vi "TCP_TB.vi"(4 "IP ADDRESS":string="192.168.0.100", 5 "error in (no error)":errorcluster, 6 "COMMAND":string, 8 "Connection ID IN":refnum<k5>) -> (0 "error out":errorcluster, 2 "Decimal Number":u32, 3 "Their Response:":string)   [LabVIEW 2013]
panel:
  out "Connection ID IN 2":refnum<k5>
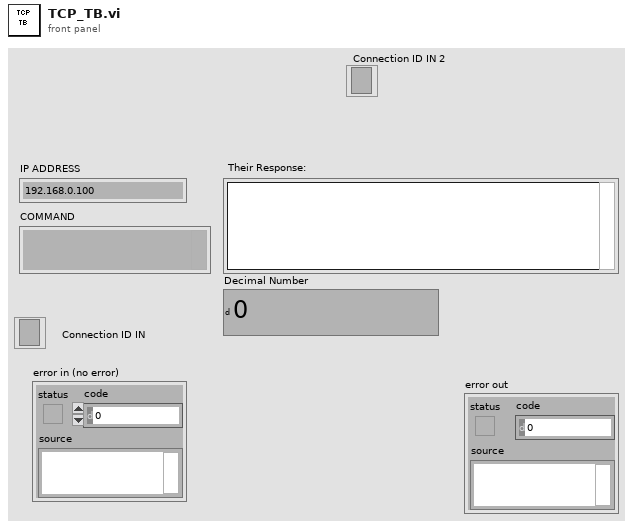
[diagram p1: front panel]
types:
  T1 = enum16{"Standard", "Buffered", "CRLF", "Immediate"}
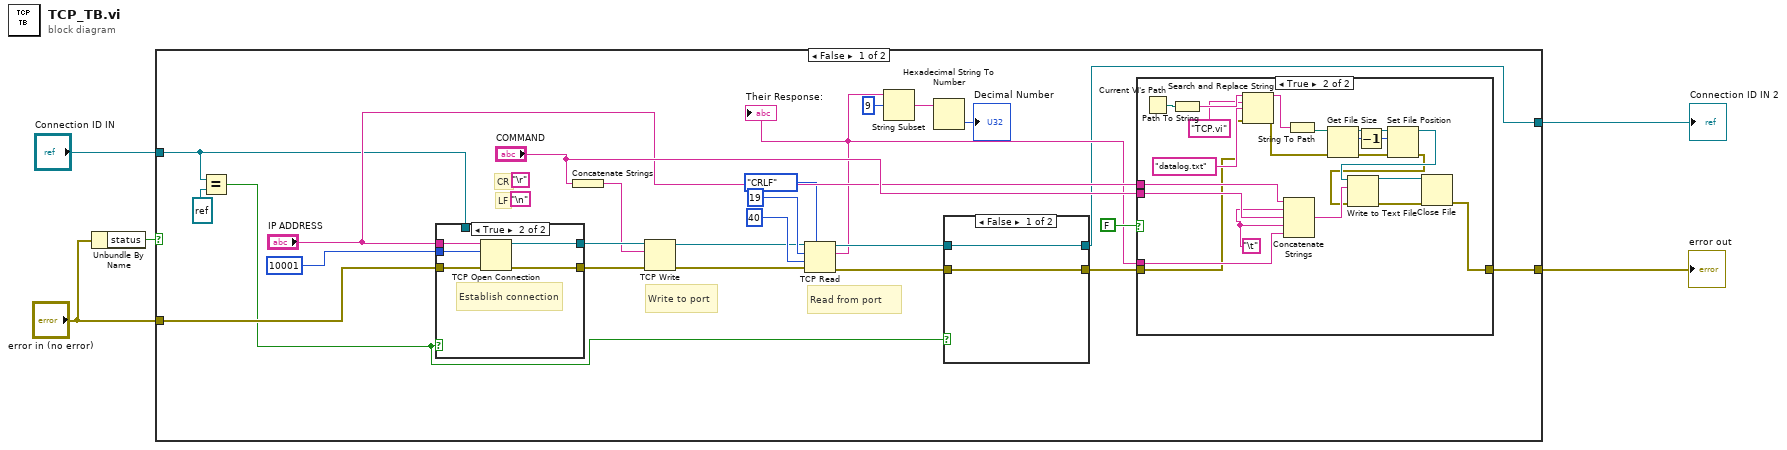
[diagram p0: block diagram]
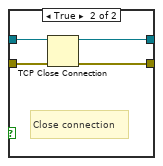
[diagram p3: hidden frame]
diagram:
  n1 = Unbundle By Name("error in (no error)") -> ("status"=w3:bool)
  n2 = case shown="False" w3 {
    tunnel: [w18 w68] -> w5
    tunnel: "error in (no error)" -> [w17 w68]
    tunnel: "Connection ID IN" -> [w9 w67]
    tunnel: [w6 w67] -> w1
    frame False {
      (unwired) "\n"
      (unwired) "\r"
      # "Read from port"
      # "Write to port"
      # "LF"
      # "CR"
      n3 = Equal?(x=w9, y=refnum<k5> refnum ("connection ID")) -> (x = y?=w7:bool)
      n4 = case shown="True" w7 {
        tunnel: [w31 w37] -> w27
        tunnel: [w32 w36] -> w26
        tunnel: u16 10001 ("remote port") -> [_ w35]
        tunnel: "IP ADDRESS" -> [_ w34]
        tunnel: w17 -> [w31 w33]
        tunnel: w9 -> [w32 _]
        frame False {
        }
        frame True {
          # "Establish connection"
          n5 = TCP Open Connection(address=w34, remote port or service name=w35, error in (no error)=w33) -> (connection ID=w36:refnum<k5>, error out=w37:errorcluster)  [unwired: 2 in]
        }
      }
      n6 = Concatenate Strings("COMMAND") -> (w24:string)
      n7 = TCP Write(connection ID=w26, data in=w24, error in (no error)=w27) -> (connection ID out=w28:refnum<k5>, error out=w16:errorcluster)  [unwired: 1 in, 1 out]
      n8 = TCP Read(connection ID=w28, bytes to read=19, error in (no error)=w16, 7:T1."CRLF" ("mode (standard)"), 9:40) -> (connection ID out=w25:refnum<k5>, data out=w13:string, error out=w15:errorcluster)
      "Their Response:" <- w13
      n9 = String Subset(string=w13, offset (0)=9) -> (substring=w14:string)  [unwired: 1 in]
      n10 = Hexadecimal String To Number(string=w14) -> (number=→"Decimal Number":u32)  [unwired: 2 in, 1 out]
      n11 = case shown="False" w7 {
        tunnel: w25 -> [w38 w43]
        tunnel: [w39 w42] -> w19
        tunnel: w15 -> [w39 w41]
        tunnel: [w38 w40] -> w6
        frame False {
        }
        frame True {
          # "Close connection"
          n12 = TCP Close Connection(connection ID=w43, error in (no error)=w41) -> (connection ID out=w40:refnum<k5>, error out=w42:errorcluster)  [unwired: 1 in]
        }
      }
      n13 = case shown="True" FALSE {
        tunnel: "COMMAND" -> [_ w66]
        tunnel: w13 -> [_ w65]
        tunnel: "IP ADDRESS" -> [_ w51]
        tunnel: w19 -> [w44 w50]
        tunnel: [w44 w45] -> w18
        frame False {
        }
        frame True {
          w52 = "\t"
          n14 = Current VI's Path() -> (path=w62:path)
          n15 = Path To String(path=w62) -> (string=w61:string)
          n16 = Search and Replace String(input string=w61, search string="TCP.vi" ("substring (\"\")"), replace string="datalog.txt" ("name or relative path"), error in=w50) -> (result string=w58:string, error out=w49:errorcluster)  [unwired: 4 in, 2 out]
          n17 = Concatenate Strings(w51, w52, w66, w52, w65) -> (w64:string)
          n18 = String To Path(string=w58) -> (path=w55:path)
          n19 = Get File Size(file=w55, error in=w49) -> (refnum out=w56:refnum<file>, size (in bytes)=w57:i64, 0:w48:errorcluster)
          n20 = Decrement(x=w57) -> (x-1=w53:i64)
          n21 = Set File Position(offset (in bytes) (0)=w53, refnum=w56, error in=w48) -> (refnum out=w54:refnum<file>, error out=w47:errorcluster)  [unwired: 1 in]
          n22 = Write to Text File(file (use dialog)=w54, text=w64, error in=w47) -> (refnum out=w63:refnum<file>, error out=w46:errorcluster)  [unwired: 1 in, 1 out]
          n23 = Close File(refnum=w63, error in=w46) -> (error out=w45:errorcluster)  [unwired: 1 out]
        }
      }
    }
    frame True {
    }
  }
  "error out" <- w5
  "Connection ID IN 2" <- w1
